vi "[RT] eHS Signal Routing.vi"(8 "Error In":errorcluster, 9 "eHS Input Mapping Keys":T4[](array[typedef]), 10 "eHS Switch Mapping Keys":T1[](array[typedef])=[{"Switch Source Types"=enum."Group B", "Source Index"=0, "Invert?"=FALSE}, {"Switch Source Types"=enum."Group B", "Source Index"=1, "Invert?"=FALSE}, {"Switch Source Types"=enum."Group B", "Source Index"=2, "Invert?"=FALSE}, {"Switch Source Types"=enum."Group B", "Source Index"=3, "Invert?"=FALSE}, {"Switch Source Types"=enum."Group B", "Source Index"=4, "Invert?"=FALSE}, {"Switch Source Types"=enum."Group B", "Source Index"=5, "Invert?"=FALSE}], 11 "FPGA VI Reference In":T3) -> (0 "Error Out":errorcluster, 3 "FPGA VI Reference Out":T3)   [LabVIEW 2017]
uses:
  Controls/eHS FPGA Ref.ctl
  <vilib>/OPAL-RT/Utilities Toolkit/Mapping/Input Mapping/Common/Controls/Input Mapping Parameters.ctl
  <vilib>/OPAL-RT/Utilities Toolkit/Mapping/Input Mapping/Common/Controls/Input Source Types.ctl
  <vilib>/OPAL-RT/Utilities Toolkit/Mapping/Switch Mapping/Common/Controls/Switch Mapping Parameters.ctl
  <vilib>/OPAL-RT/Utilities Toolkit/Mapping/Switch Mapping/Common/Controls/Switch Source Types.ctl
  <vilib>/OPAL-RT/Utilities Toolkit/Mapping/Input Mapping/Host/Controls/Number of Inputs.ctl
  <vilib>/OPAL-RT/Utilities Toolkit/Mapping/Switch Mapping/Host/Controls/Number of Switches.ctl
  <vilib>/OPAL-RT/Utilities Toolkit/Mapping/Input Mapping/Host/SubVIs/Pack & Send Input Mapping Configuration to Target.vi
  <vilib>/OPAL-RT/Utilities Toolkit/Mapping/Switch Mapping/Host/SubVIs/Pack & Send Switch Mapping Configuration to Target.vi
  <vilib>/OPAL-RT/Utilities Toolkit/Mapping/Input Mapping/Host/Input Mapping - Host.lvlib
  <vilib>/OPAL-RT/Utilities Toolkit/Mapping/Switch Mapping/Host/Switch Mapping - Host.lvlib
  <vilib>/OPAL-RT/Utilities Toolkit/Mapping/Input Mapping/Common/Input Mapping - Common.lvlib
  <vilib>/OPAL-RT/Utilities Toolkit/Mapping/Switch Mapping/Common/Switch Mapping - Common.lvlib
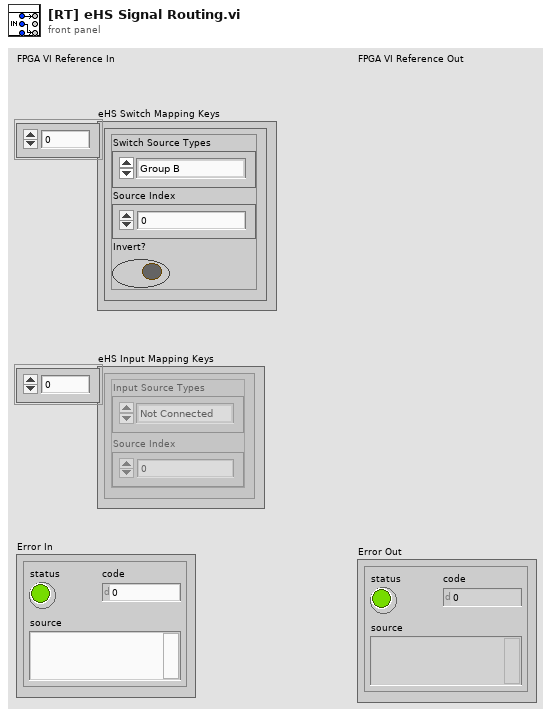
[diagram p1: front panel]
types:
  T1 = typedef "Switch Mapping - Common.lvlib/Switch Mapping Parameters.ctl" = cluster{"Switch Source Types":T2, "Source Index":u8, "Invert?":bool}
  T2 = typedef "Switch Mapping - Common.lvlib/Switch Source Types.ctl" = enum16{"Not Connected", "Group A", "Group B", "Group C", "Group D", "Group E"}
  T3 = typedef "eHS FPGA Ref.ctl" = refnum<k20>
  T4 = typedef "Input Mapping - Common.lvlib/Input Mapping Parameters.ctl" = cluster{"Source Index":u8, "Input Source Types":T5}
  T5 = typedef "Input Mapping - Common.lvlib/Input Source Types.ctl" = enum16{"Not Connected", "Group A", "Group B", "Group C", "Group D"}
  T6 = typedef "Switch Mapping - Host.lvlib/Number of Switches.ctl" = enum16{"72"}
  T7 = typedef "Input Mapping - Host.lvlib/Number of Inputs.ctl" = enum16{"32"}
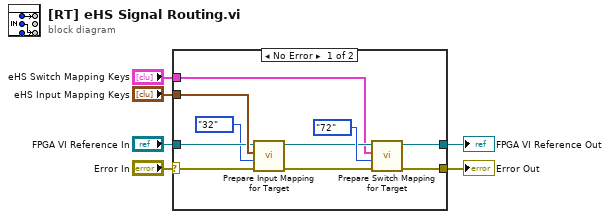
[diagram p0: block diagram]
diagram:
  n1 = case shown="No Error" "Error In" {
    selector: "Error In" -> [w8 w18]
    tunnel: "eHS Input Mapping Keys" -> [w16 _]
    tunnel: "FPGA VI Reference In" -> [w15 w17]
    tunnel: [w10 w17] -> w4
    tunnel: [w9 w18] -> w3
    tunnel: "eHS Switch Mapping Keys" -> [w7 _]
    frame No Error {
      n2 = call-poly <vilib>:"Prepare Input Mapping for Target.vi"("Error In"=w8, "Number of Inputs"=Number_of_Inputs."32", "Input Mapping Keys"=w16, "FPGA VI Reference In"=w15) -> ("Error Out"=w11:errorcluster, "FPGA VI Reference Out"=w12:T3)  [unwired: 6 in]
      n3 = call-poly <vilib>:"Prepare Switch Mapping for Target .vi"("Error In"=w11, "#Switches"=Number_of_Switches."72", "Switch Mapping Keys"=w7, "FPGA VI Reference In"=w12) -> ("Error Out"=w9:errorcluster, "FPGA VI Reference Out"=w10:T3)  [unwired: 6 in]
    }
    frame Error {
    }
  }
  "Error Out" <- w3
  "FPGA VI Reference Out" <- w4
